vi "Read Data to Encode.vi"(8 "error in (no error)":errorcluster) -> (0 "error out":errorcluster, 3 "Data to Encode":string)   [LabVIEW 2014]
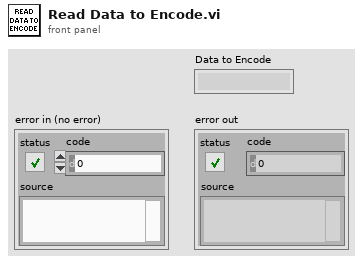
[diagram p1: front panel]
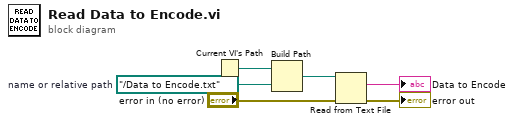
[diagram p0: block diagram]
diagram:
  w5 = path "../Data to Encode.txt"  # name or relative path
  n1 = Current VI's Path() -> (path=w6:path)
  n2 = Build Path(base path=w6, name or relative path=w5) -> (appended path=w4:path)
  n3 = Read from Text File(file (use dialog)=w4, error in="error in (no error)") -> (text=→"Data to Encode":string, error out=→"error out":errorcluster)  [unwired: 2 in, 2 out]
